vi "Check - Inherit from QControl.vi"(11 "New QControl Info":refnum<data-value>) -> (0 "error out":errorcluster)   [LabVIEW 2019, in "New QControl Info.lvclass"]
doc: "<b> </b> <b> </b>\n©2016 Q Software Innovations, LLC (QSI)\nwritten by Quentin Alldredge\nproduced in LabVIEW 2015\n\nsupport@qsoftwareinnovations.com\nwww.qsoftwareinnovations.com\n\nAll rights reserved.\n\nRedistribution and use in source and binary forms, with or without modification, are permitted provided that the following conditions are met:\n\n * Redistributions of source code must retain the above copyright notice, this list of conditions and the following disclaimer.\n * Redistributions in binary form must reproduce the above copyright notice, this list of conditions and the following disclaimer in the documentation and/or other materials provided with the distribution.\n * Neither the name of Q Software Innovations, LLC. nor the names of its contributors may be used to endorse or promote products derived from this software without specific prior written permission.\n\nTHIS SOFTWARE IS PROVIDED BY THE COPYRIGHT HOLDERS AND CONTRIBUTORS \"AS IS\" AND ANY EXPRESS OR IMPLIED WARRANTIES, INCLUDING, BUT NOT LIMITED TO, THE IMPLIED WARRANTIES OF MERCHANTABILITY AND FITNESS FOR A PARTICULAR PURPOSE ARE DISCLAIMED. IN NO EVENT SHALL THE COPYRIGHT OWNER OR CONTRIBUTORS BE LIABLE FOR ANY DIRECT, INDIRECT, INCIDENTAL, SPECIAL, EXEMPLARY, OR CONSEQUENTIAL DAMAGES (INCLUDING, BUT NOT LIMITED TO, PROCUREMENT OF SUBSTITUTE GOODS OR SERVICES; LOSS OF USE, DATA, OR PROFITS; OR BUSINESS INTERRUPTION) HOWEVER CAUSED AND ON ANY THEORY OF LIABILITY, WHETHER IN CONTRACT, STRICT LIABILITY, OR TORT (INCLUDING NEGLIGENCE OR OTHERWISE) ARISING IN ANY WAY OUT OF THE USE OF THIS SOFTWARE, EVEN IF ADVISED OF THE POSSIBILITY OF SUCH DAMAGE."
uses:
  New QControl Info/New QControl Info.lvclass
  QControl Classes/Control/Control.lvclass
  New QControl Info/New QControl Info.lvclass/New QControl Info.ctl
  New QControl Info/Read Parent Class Path.vi
  New QControl Info/Read App Refnum.vi
  <vilib>/ErrorRing/Error Ring.xnode
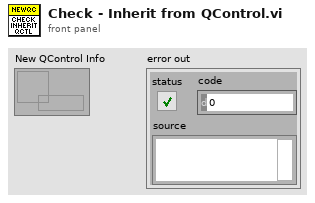
[diagram p1: front panel]
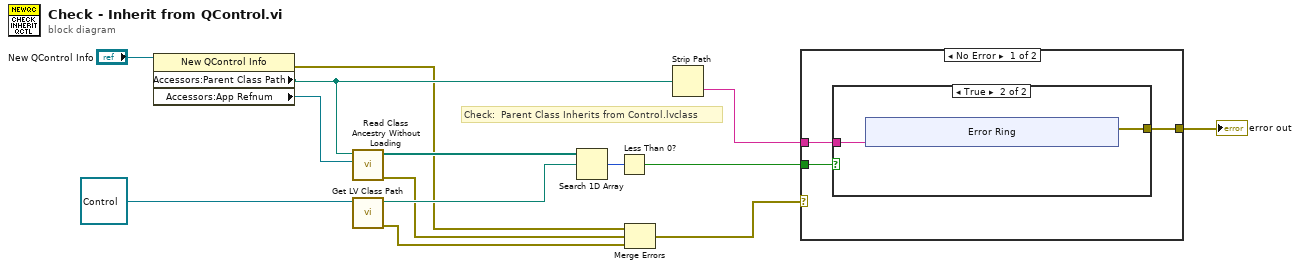
[diagram p0: block diagram]
diagram:
  # "Check:  Parent Class Inherits from Control.lvclass"
  n1 = property class="New QControl Info"(reference="New QControl Info") -> (error out=w4:errorcluster, "Accessors:Parent Class Path"=w6:path, "Accessors:App Refnum"=w5:refnum<vi>)  [unwired: 1 in, 1 out]
  n2 = call <vilib>:"Read Class Ancestry Without Loading.vi"("App Reference (this app)"=w5, "LabVIEW Class Path"=w6) -> ("error out"=w3:errorcluster, "Class Ancestry"=w12:path[])  [unwired: 8 in]
  n3 = call <vilib>:"Get LV Class Path.vi"("object"=refnum<class "Control.lvclass"> refnum ("Control")) -> ("error out"=w2:errorcluster, "class path"=w13:path)  [unwired: 9 in]
  n4 = Search 1D Array(1D array=w12, element=w13) -> (index of element=w14:i32)  [unwired: 1 in]
  n5 = Less Than 0?(x=w14) -> (x < 0?=w9:bool)
  n6 = Merge Errors(w4, w3, w2) -> (w1:errorcluster)
  n7 = Strip Path(path=w6) -> (name=w10:string)  [unwired: 1 out]
  n8 = case shown="No Error" w1 {
    selector: w1 -> [_ w25]
    tunnel: w10 -> [w17 _]
    tunnel: w9 -> [w16 _]
    tunnel: [w15 w25] -> w8
    frame No Error {
      n9 = case shown="True" w16 {
        tunnel: w17 -> [_ w19]
        tunnel: [_ w18] -> w15
        frame False {
        }
        frame True {
          n10 = xnode "Error Ring"("parameter 0"=w19) -> ("error out"=w18:errorcluster)
        }
      }
    }
    frame Error {
    }
  }
  "error out" <- w8
